vi "Main.vi"(5 "Run_Popup":bool, 7 "Stop":bool, 9 "Wait":bool, 11 "error in":T1) -> (4 "error out":T2)   [LabVIEW 2020]
doc: "This VI is used to do some basic controls on the sub VI with the help of invoke node"
uses:
  Typedefs/Errorin.ctl
  Typedefs/Errorout.ctl
panel:
  # "VI to open the front panel of another vi and controlling it"
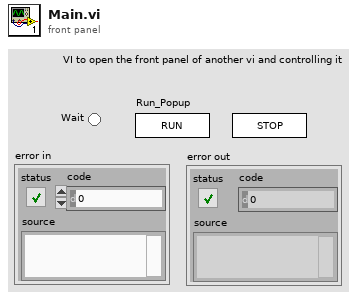
[diagram p1: front panel]
types:
  T1 = typedef "Errorin.ctl" = errorcluster
  T2 = typedef "Errorout.ctl" = errorcluster
  T3 = enum8{"Enabled", "Disabled", "Disabled and Grayed Out"}
  T4 = enum32{"Bad", "Idle", "Run top level", "Running"}
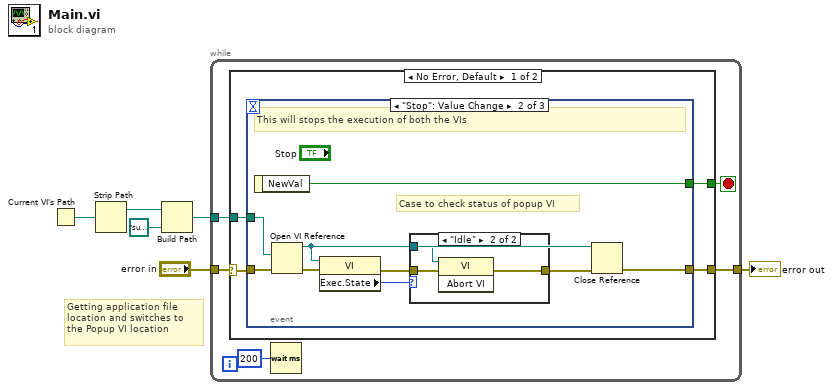
[diagram p0: block diagram]
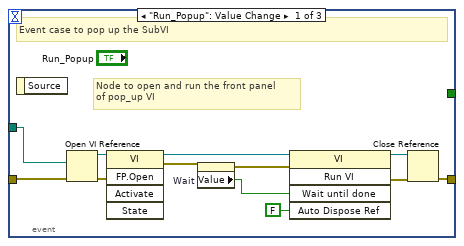
[diagram p2: hidden frame]
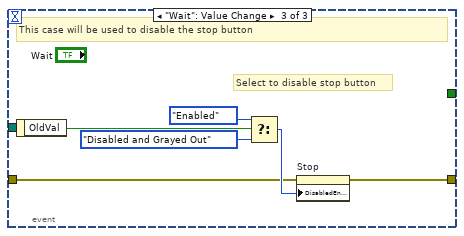
[diagram p4: hidden frame]
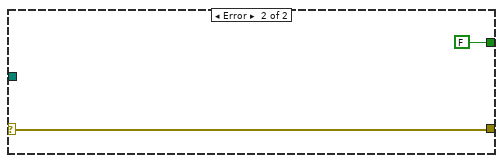
[diagram p5: hidden frame]
diagram:
  # "Getting application file \nlocation and switches to \nthe Popup VI location"
  n1 = Current VI's Path() -> (path=w4:path)
  n2 = Strip Path(path=w4) -> (stripped path=w3:path)  [unwired: 1 out]
  n3 = Build Path(base path=w3, name or relative path=path "subVI/Pop_up.vi") -> (appended path=w5:path)
  n4 = while {
    tunnel: w5 -> [w10]
    tunnel: "error in" -> [w7]
    tunnel: [w8] -> w1
    stop <- w11 stop-if-true
    n5 = case shown="No Error, Default" w7 {
      selector: w7 -> [w12 w46]
      tunnel: [w15 FALSE ("NewVal")] -> w11
      tunnel: w10 -> [w14 _]
      tunnel: [w13 w46] -> w8
      frame No Error {
        n6 = event shown="[1] \"Stop\": Value Change" {
          selector: _ -> [_ _ _]
          dyn-events: _ -> [_ _ _]
          timeout: _ -> [_ _ _]
          tunnel: [_ w35 _] -> w15
          tunnel: [w22 w33 w41] -> w13
          tunnel: w12 -> [w21 w36 w40]
          tunnel: w14 -> [w20 w34 _]
          event "Run_Popup": Value Change {
            # "Node to open and run the front panel \nof pop_up VI"
            # "Event case to pop up the SubVI"
            n7 = event-data() -> ()  [unwired: 1 in, 1 out]
            n8 = Open VI Reference(vi path=w20, error in (no error)=w21) -> (vi reference=w27:refnum<vi>, error out=w23:errorcluster)  [unwired: 4 in]
            n9 = invoke class="VI" method="FP.Open"(reference=w27, error in=w23) -> (reference out=w16:refnum<vi>, error out=w19:errorcluster)  [unwired: 3 in, 3 out]
            n10 = property on="Wait" class="Bool (strict)"(error in=w19) -> (error out=w18:errorcluster, "Value"=w17:bool)  [unwired: 1 in, 1 out]
            n11 = invoke class="VI" method="Run VI"(reference=w16, error in=w18, "Wait until done"=w17, "Auto Dispose Ref"=FALSE ("Auto Dispose Reference")) -> (reference out=w26:refnum<vi>, error out=w24:errorcluster)  [unwired: 1 in, 3 out]
            n12 = Close Reference(reference=w26, error in (no error)=w24) -> (error out=w22:errorcluster)
          }
          event "Stop": Value Change {
            # "Case to check status of popup VI"
            # "This will stops the execution of both the VIs"
            n13 = event-data() -> ("NewVal"=w35:bool)  [unwired: 1 in]
            n14 = Open VI Reference(vi path=w34, error in (no error)=w36) -> (vi reference=w30:refnum<vi>, error out=w31:errorcluster)  [unwired: 4 in]
            n15 = property class="VI"(reference=w30, error in=w31) -> (error out=w32:errorcluster, "Exec.State"=w28:T4)  [unwired: 1 out]
            n16 = case shown="\"Idle\"" w28 {
              tunnel: w32 -> [_ w39]
              tunnel: w30 -> [_ w38]
              tunnel: [_ w37] -> w29
              frame "Bad", Default {
              }
              frame "Idle" {
                n17 = invoke class="VI" method="Abort VI"(reference=w38, error in=w39) -> (error out=w37:errorcluster)  [unwired: 1 in, 2 out]
              }
            }
            n18 = Close Reference(reference=w30, error in (no error)=w29) -> (error out=w33:errorcluster)
          }
          event "Wait": Value Change {
            # "Select to disable stop button"
            # "This case will be used to disable the stop button"
            n19 = event-data() -> ("OldVal"=w43:bool)  [unwired: 1 in]
            n20 = Select(t=T3."Enabled" ("Disabled"), s=w43, f=T3."Disabled and Grayed Out" ("Disabled")) -> (s? t:f=w42:T3)
            n21 = property on="Stop" class="Bool"(error in=w40, "DisabledEnum"=w42) -> (error out=w41:errorcluster)  [unwired: 1 in, 1 out]
          }
        }
      }
      frame Error {
      }
    }
    n22 = Wait (ms)(milliseconds to wait=u32 200) -> ()  [unwired: 1 out]
  }
  "error out" <- w1
